vi "Log Data to File.vi"(0 "Logging Data to File":bool=TRUE, 5 "File Path":path=path "c:/Temp/Data.lvm", 7 "Measurement Names":string[](array[string]), 9 "Data":dbl[](array[numeric]) format="%.2g", 11 "Error In":errorcluster) -> (15 "Error Out":errorcluster)   [LabVIEW 2018]
uses:
  <vilib>/express/express signal manip/GetorSetDDTAttributes/Shared VIs/TimeType.ctl
  <vilib>/express/express signal manip/GetorSetDDTAttributes/Shared VIs/TimeMode Enum to Boolean.vi
  <vilib>/express/express shared/transition.llb/Dynamic To Waveform Array.vi
  <vilib>/express/express signal manip/GetorSetDDTAttributes/Set DDT Attributes/SetT0.vi
  <vilib>/express/express signal manip/GetorSetDDTAttributes/Set DDT Attributes/sub Set StartTimeStamp.vi
  <vilib>/express/express shared/transition.llb/Waveform Array To Dynamic.vi
  <vilib>/express/express signal manip/GetorSetDDTAttributes/Set DDT Attributes/Set DDT Properties.xnode
  <vilib>/express/express signal manip/GetorSetDDTAttributes/Shared VIs/GetSetShared.lvlib
  <vilib>/express/express signal manip/GetorSetDDTAttributes/Set DDT Attributes/Set DDT Attributes.lvlib
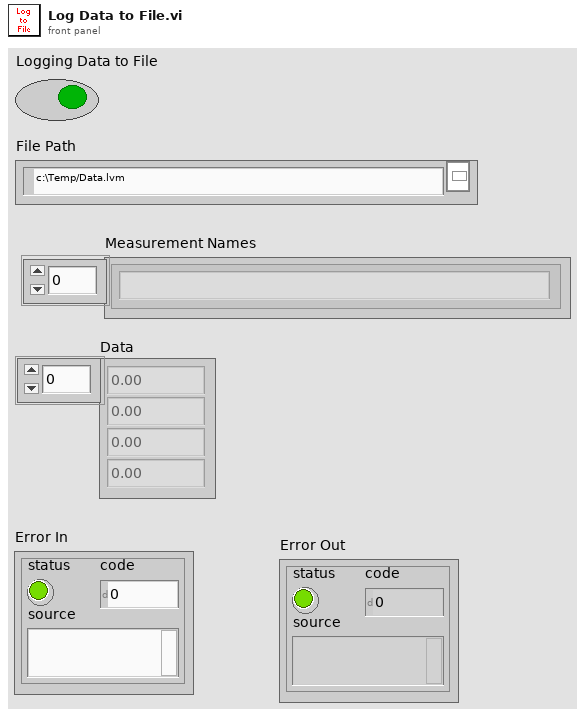
[diagram p1: front panel]
types:
  T1 = typedef "GetSetShared.lvlib/TimeType.ctl" = enum16{"Absolute", "Relative"}
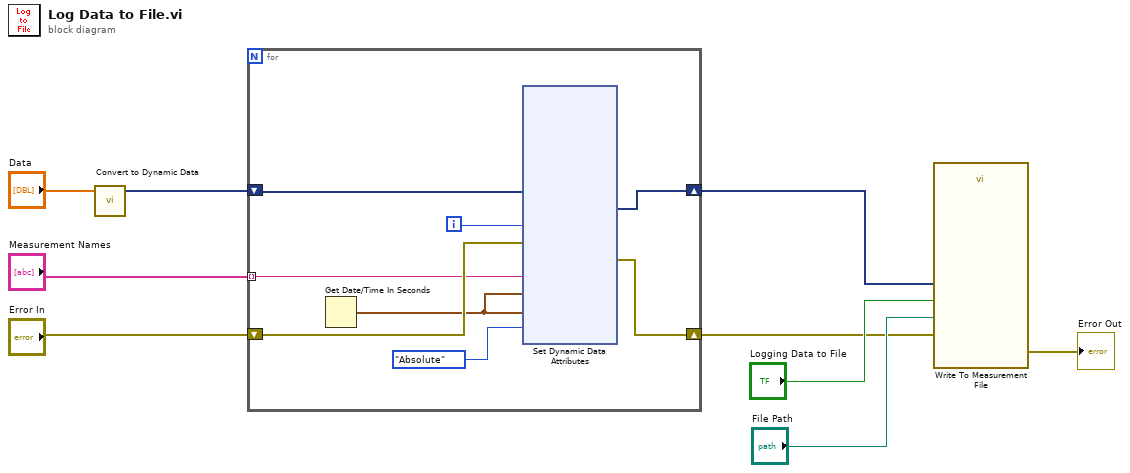
[diagram p0: block diagram]
diagram:
  n1 = call "Convert to Dynamic Data"("Array"="Data") -> ("Dynamic Data Type"=w3:dynamicdata)  [unwired: 3 in]
  n2 = for {
    shift-right: [w16] -> w6
    shift-left: "Error In" -> [w17]
    shift-right: [w12] -> w1
    shift-left: w3 -> [w13]
    tunnel: "Measurement Names" -> [w11] mode=indexing
    i -> [w10]
    n3 = Get Date/Time In Seconds() -> (seconds since 1Jan1904=w15:timestamp)
    n4 = xnode "Set Dynamic Data Attributes"("Signals In"=w13, "Signal Index"=w10, "error in"=w17, "Signal Name"=w11, "Start Timestamp"=w15, "Timestamp"=w15, "Time Mode"=TimeType."Absolute") -> ("Signals Out"=w12:dynamicdata, "error out"=w16:errorcluster)
  }
  n5 = call "Write To Measurement File"("Signals"=w1, "Enable"="Logging Data to File", "error in (no error)"=w6, "Filename"="File Path") -> ("error out"=→"Error Out":errorcluster)  [unwired: 13 in, 2 out]
